vi "SetPersistentConfiguration.vi"(8 "Error In":errorcluster, 9 "DataIn":variant, 11 "object in":refnum<class "IPersistentData.lvclass">) -> (0 "Error Out":errorcluster, 1 "DataOut":variant, 3 "object out":refnum<class "IPersistentData.lvclass">)   [LabVIEW 2021, in "IPersistentData.lvclass"]
uses:
  IPersistentData.lvclass
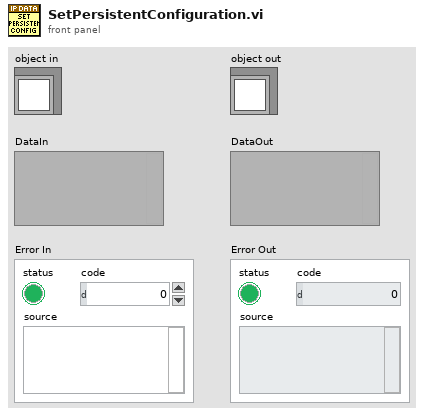
[diagram p1: front panel]
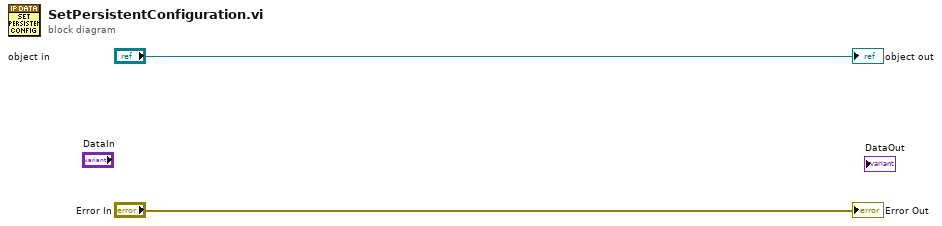
[diagram p0: block diagram]
diagram:
  "Error Out" <- "Error In"
  "object out" <- "object in"
